vi "Icon_2D color to 1D.vi"(8 "Error":errorcluster, 11 "2D Image":T1) -> (0 "Error Out":errorcluster, 1 "Sorted By Quantity Out":u32[](array[colorbox]), 3 "1D Array Out":u32[](array[colorbox]))   [LabVIEW 2009]
doc: "Transforms the 2D Image to 1D color array and sorts base on size"
uses:
  Controls/Array/Color Box Array_2D Icon Viewer.ctl
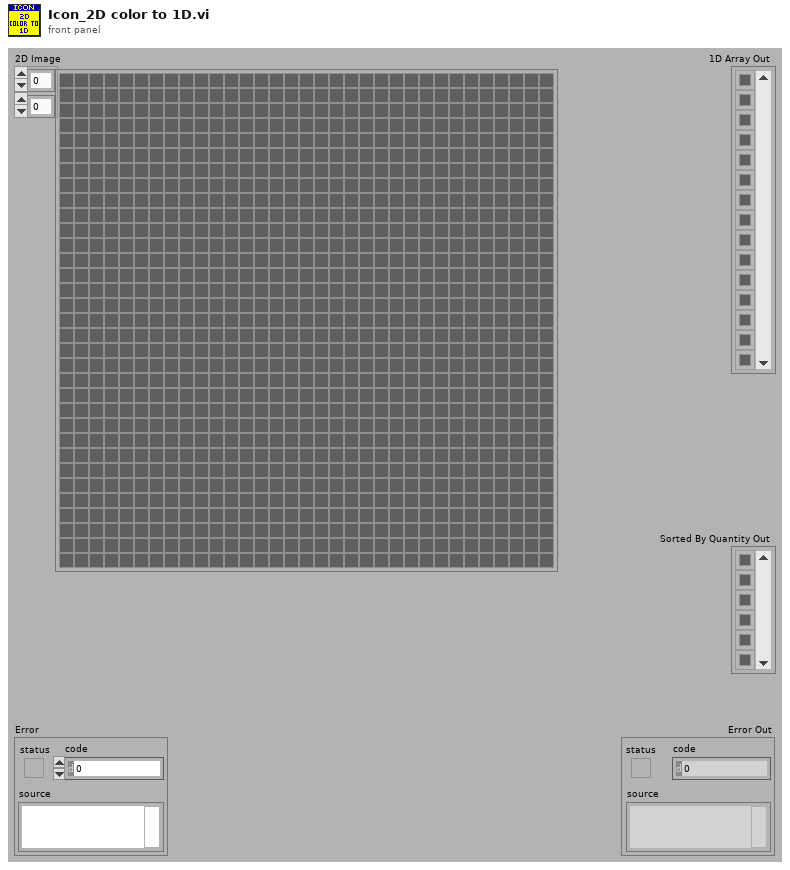
[diagram p1: front panel]
types:
  T1 = typedef "Color Box Array_2D Icon Viewer.ctl" = u32[][]
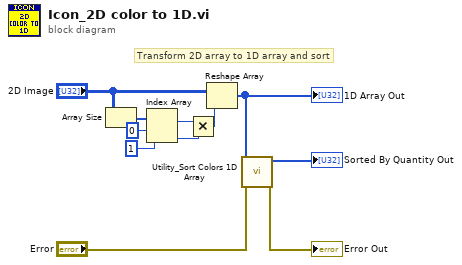
[diagram p0: block diagram]
diagram:
  # "Transform 2D array to 1D array and sort"
  n1 = Array Size(array="2D Image") -> (size(s)=w8:i32[])
  n2 = Index Array(array=w8, index #1=0 ("index"), index #2=1 ("index")) -> (element #1=w9:i32, element #2=w10:i32)
  n3 = Multiply(x=w9, y=w10) -> (x*y=w11:i32)
  n4 = Reshape Array("2D Image", w11) -> (w4:u32[])
  "1D Array Out" <- w4
  n5 = call "Utility_Sort Colors 1D Array.vi"("Error"="Error", "Colors"=w4) -> ("Error Out"=→"Error Out":errorcluster, "Sorted By Quantity Out"=→"Sorted By Quantity Out":u32[])  [unwired: 7 in, 1 out]
